vi "Configuration Session Test.vi"   [LabVIEW 2017]
uses:
  Classes/Configuration/Configuration Session.lvclass
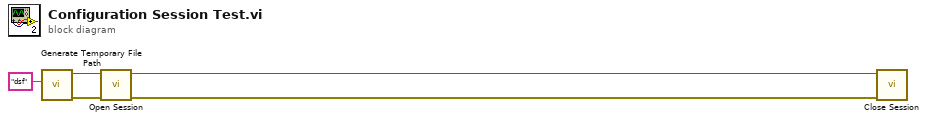
[diagram p0: block diagram]
diagram:
  n1 = call <vilib>:"Generate Temporary File Path.vi"("Temporary File Extension (tmp)"="dsf") -> ("error out"=w3:errorcluster, "Unique Temporary File Path"=w4:path)  [unwired: 9 in]
  n2 = call "Open Session.vi"("error in (no error)"=w3, "configuration file path"=w4) -> ("error out"=w1:errorcluster, "configuration session"=w2:refnum<class "Configuration Session.lvclass">)  [unwired: 5 in, 3 out]
  n3 = call "Close Session.vi"("error in (no error)"=w1, "configuration session"=w2) -> ()  [unwired: 8 in, 2 out]
